vi "SetCurvesParams.vi"(8 "error in (no error)":errorcluster caption="entrée d'erreur (pas d'erreur)", 10 "CurvesParams":T1[](array[typedef]), 11 "Interface en entrée":refnum<class "Interface.lvclass">) -> (0 "error out":errorcluster caption="sortie d'erreur", 3 "Interface en sortie":refnum<class "Interface.lvclass">)   [LabVIEW 2010, in "Interface.lvclass"]
uses:
  Interface.lvclass
  CurveParams.ctl
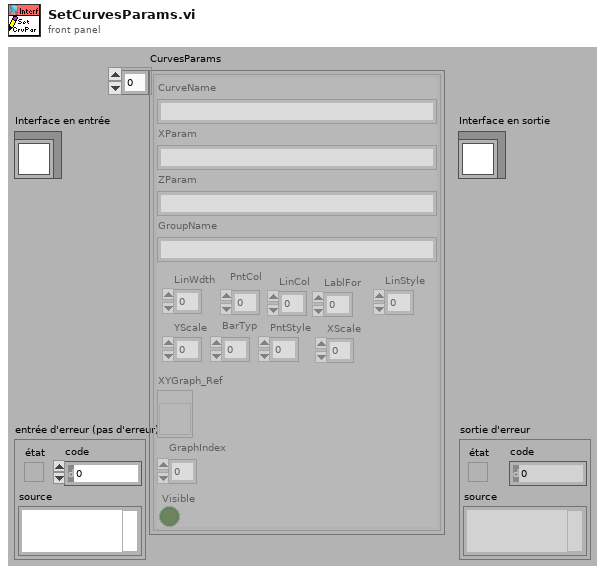
[diagram p1: front panel]
types:
  T1 = typedef "Interface.lvclass/CurveParams.ctl" = cluster{"CurveName":string, "XParam":string, "ZParam ":string, "GroupName":string, "BarTyp":u8, "LinWdth":u32, "LinStyle":u32, "XYGraph_Ref":refnum<vi>, "GraphIndex":i32, "Visible":bool, "PntCol":u8, "PntStyle":u32, "LinCol":u8, "LablFor":u8, "XScale":u32, "YScale":u32}
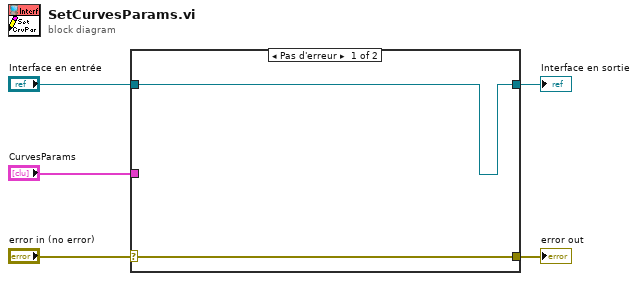
[diagram p0: block diagram]
diagram:
  n1 = case shown="Pas d'erreur" "error in (no error)" {
    selector: "error in (no error)" -> [w7 w8]
    tunnel: [w7 w8] -> w4
    tunnel: [w6 w9] -> w2
    tunnel: "Interface en entrée" -> [w6 w9]
    tunnel: "CurvesParams" -> [_ _]
    frame No Error {
    }
    frame Error {
    }
  }
  "error out" <- w4
  "Interface en sortie" <- w2
